vi "ReadSingleEvent.vi"(0 "InputEventWord":u32[](array[numeric])) -> (3 "ChipID":u16 format="%x", 4 "TimeSamp":u64, 6 "PixelAddress":u32, 8 "TDCValue":u32, 10 "TemperatureValue":u32, 14 "ADCTrigPix":u32, 15 "ADCPixels":u32[](array[numeric]))   [LabVIEW 2015, in "VIPM2.lvlib"]
uses:
  VIPM2.lvlib
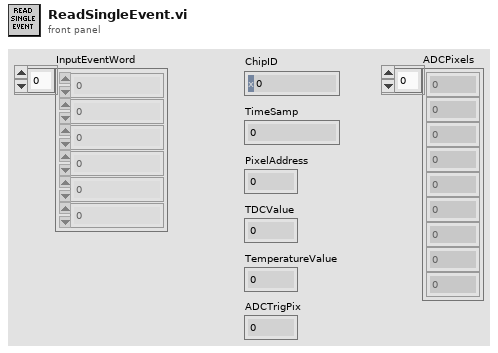
[diagram p1: front panel]
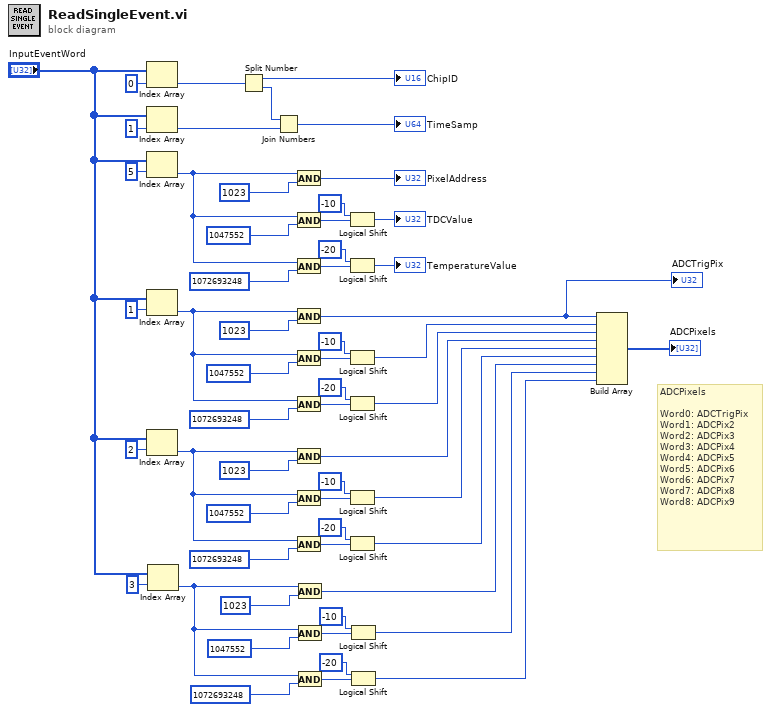
[diagram p0: block diagram]
diagram:
  # "ADCPixels\n\nWord0: ADCTrigPix\nWord1: ADCPix2\nWord2: ADCPix3\nWord3: ADCPix4\nWord4: ADCPix5\nWord5: ADCPix6\nWord6: ADCPix7\nWord7: ADCPix8\nWord8: ADCPix9"
  n1 = Index Array(array="InputEventWord", index=0) -> (element=w57:u32)
  n2 = Index Array(array="InputEventWord", index=1) -> (element=w52:u32)
  n3 = Index Array(array="InputEventWord", index=5) -> (element=w40:u32)
  n4 = Index Array(array="InputEventWord", index=1) -> (element=w37:u32)
  n5 = Index Array(array="InputEventWord", index=2) -> (element=w22:u32)
  n6 = Index Array(array="InputEventWord", index=3) -> (element=w19:u32)
  n7 = Split Number(x=w57) -> (hi(x)=→"ChipID":u16, lo(x)=w53:u16)
  n8 = Join Numbers(hi=w53, lo=w52) -> ((hi.lo)=→"TimeSamp":u64)
  n9 = And(x=w40, y=u32 1023) -> (x .and. y?=→"PixelAddress":u32)
  n10 = And(x=w40, y=u32 1047552) -> (x .and. y?=w46:u32)
  n11 = And(x=w40, y=u32 1072693248) -> (x .and. y?=w42:u32)
  n12 = And(x=w37, y=u32 1023) -> (x .and. y?=w10:u32)
  "ADCTrigPix" <- w10
  n13 = And(x=w37, y=u32 1047552) -> (x .and. y?=w33:u32)
  n14 = And(x=w37, y=u32 1072693248) -> (x .and. y?=w35:u32)
  n15 = And(x=w22, y=u32 1023) -> (x .and. y?=w7:u32)
  n16 = And(x=w22, y=u32 1047552) -> (x .and. y?=w26:u32)
  n17 = And(x=w22, y=u32 1072693248) -> (x .and. y?=w24:u32)
  n18 = And(x=w19, y=u32 1023) -> (x .and. y?=w4:u32)
  n19 = And(x=w19, y=u32 1047552) -> (x .and. y?=w15:u32)
  n20 = And(x=w19, y=u32 1072693248) -> (x .and. y?=w17:u32)
  n21 = Logical Shift(y=i16 -10, x=w46) -> (x << y=→"TDCValue":u32)
  n22 = Logical Shift(y=i16 -20, x=w42) -> (x << y=→"TemperatureValue":u32)
  n23 = Logical Shift(y=i16 -10, x=w33) -> (x << y=w9:u32)
  n24 = Logical Shift(y=i16 -20, x=w35) -> (x << y=w8:u32)
  n25 = Logical Shift(y=i16 -10, x=w26) -> (x << y=w6:u32)
  n26 = Logical Shift(y=i16 -20, x=w24) -> (x << y=w5:u32)
  n27 = Logical Shift(y=i16 -10, x=w15) -> (x << y=w3:u32)
  n28 = Logical Shift(y=i16 -20, x=w17) -> (x << y=w2:u32)
  n29 = Build Array(w10, w9, w8, w7, w6, w5, w4, w3, w2) -> (→"ADCPixels":u32[])
